vi "ProportionalSub.vi"(11 "Bytes Read":u8[](array[numeric])) -> (1 "Numeric":dbl, 2 "y":i32, 3 "x":i32, 4 "Numeric 2":dbl)   [LabVIEW 2018]
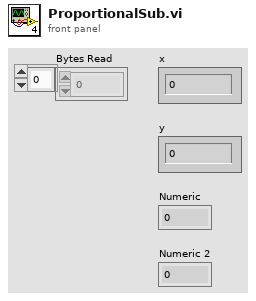
[diagram p1: front panel]
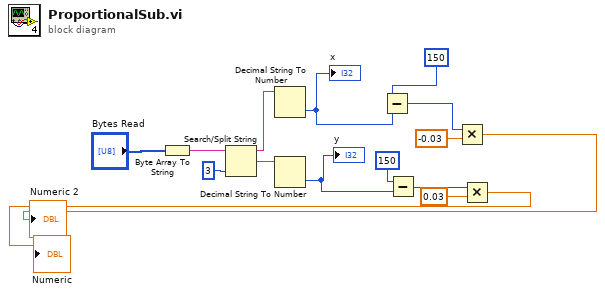
[diagram p0: block diagram]
diagram:
  n1 = Byte Array To String(unsigned byte array="Bytes Read") -> (string=w2:string)
  n2 = Search/Split String(string=w2, offset (0)=3) -> (substring before match=w4:string, match + rest of string=w5:string)  [unwired: 1 in, 1 out]
  n3 = Decimal String To Number(string=w4) -> (number=w13:i32)  [unwired: 2 in, 1 out]
  "x" <- w13
  n4 = Decimal String To Number(string=w5) -> (number=w14:i32)  [unwired: 2 in, 1 out]
  "y" <- w14
  n5 = Subtract(x=150 ("y"), y=w13) -> (x-y=w6:i32)
  n6 = Subtract(x=150 ("y"), y=w14) -> (x-y=w9:i32)
  n7 = Multiply(x=w6, y=-0.03) -> (x*y=→"Numeric 2":dbl)
  n8 = Multiply(x=w9, y=0.03) -> (x*y=→"Numeric":dbl)
